vi "Read Fetch Timeout.vi"(8 "error in (no error)":errorcluster, 11 "Fetch Waveforms CFG in":refnum<class "Fetch Waveforms CFG.lvclass">) -> (0 "error out":errorcluster, 2 "Fetch Timeout":dbl=10.0, 3 "Fetch Waveforms CFG out":refnum<class "Fetch Waveforms CFG.lvclass">)   [LabVIEW 2023, in "PXIe-4353.lvlib" / "Fetch Waveforms CFG.lvclass"]
uses:
  Fetch Waveforms CFG.lvclass
  Fetch Waveforms CFG.lvclass/Fetch Waveforms CFG.ctl
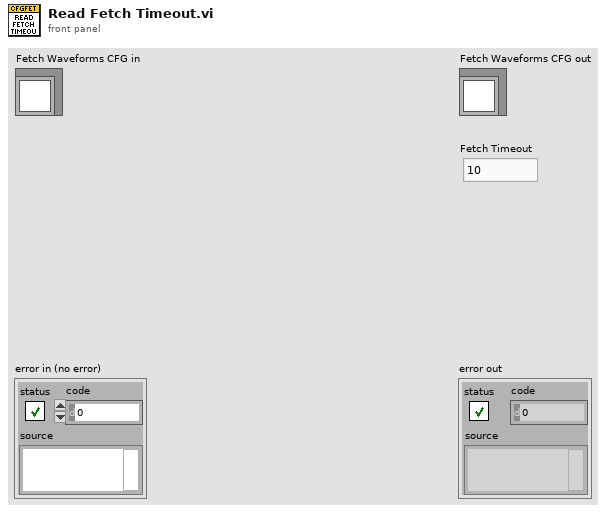
[diagram p1: front panel]
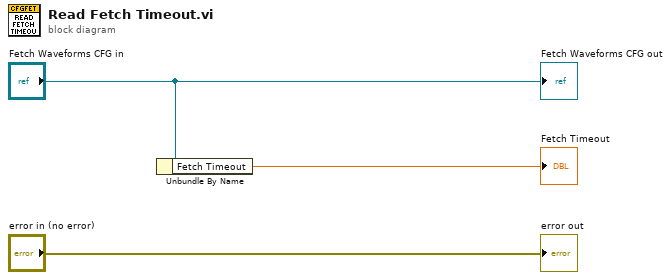
[diagram p0: block diagram]
diagram:
  n1 = Unbundle By Name("Fetch Waveforms CFG in") -> ("Fetch Timeout"=→"Fetch Timeout":dbl)
  "error out" <- "error in (no error)"
  "Fetch Waveforms CFG out" <- "Fetch Waveforms CFG in"
